vi "Purge uService from local lists.vi"(10 "Last Ack":refnum<class "Last Ack.lvclass">, 11 "Guardian in":refnum<class "Guardian.lvclass">) -> (0 "error out":errorcluster, 1 "uService ID":string, 2 "uService Properties":T1, 3 "Guardian out":refnum<class "Guardian.lvclass">)   [LabVIEW 2026, in "TALOS.lvlib" / "Guardian.lvlib" / "Guardian.lvclass"]
uses:
  Guardian.lvclass
  Classes/uService List/uService Properties.ctl
  builds/Actor Framework PPL/Actor Framework.lvlibp/1abvi3w/vi.lib/ActorFramework/Message Enqueuer/Message Enqueuer.lvclass
  C:/LabVIEW Code/TALOS/talos/Ancestor/Ancestor/Ancestor.lvclass
  builds/Actor Framework PPL/Actor Framework.lvlibp/1abvi3w/vi.lib/ActorFramework/LastAck/Last Ack.lvclass
  Classes/uService List/uService List.lvclass/uService List.ctl
  Ancestor/Ancestor/Ancestor.lvclass/Ancestor.ctl
  Classes/uService List/Get ID from Queue.vi
  Classes/uService List/Get Properties.vi
  Classes/uService List/Remove uService.vi
  Ancestor/Ancestor/Write uS List Ref.vi
  Ancestor/Ancestor/Read Distr uS Map ref.vi
  Ancestor/Ancestor/Read ID.vi
  Ancestor/Ancestor/Write Distr uS Map ref.vi
  Support VIs/Generate Error.vi
  FGV/Error Memory/Get Error Description.vi
  Support VIs/Get PC name.vi
  Support VIs/Get Class Name.vi
  <vilib>/Utility/error.llb/Clear Errors.vi
  FGV/Error Memory/Error Memory Core.vi
  <vilib>/AdvancedString/Delimited String to 1D String Array.vi
  <vilib>/AdvancedString/Delimited String to 1D String Array (string).vi
  Support VIs/Circus Root Path.vi
  FGV/Error Memory/Error Crt Lvl checker.vi
  FGV/Error Memory/Error Memory Core.vi/40c8088d-b597-4017-91af-faa98e00292e.vi
  FGV/Error Memory/Error Memory Core.vi/d4a3ab98-063c-4e44-b43d-fbdcfe6c2be2.vi
  Support VIs/Global Memory.vi
  <vilib>/Utility/LVClass/Get LV Class Name.vi
  Support VIs/Is in Packed Library.vi
  Support VIs/TALOS Root path.vi
  Support VIs/Read CSV worksheet.vi
  Support VIs/Global Constants.vi
  <vilib>/Utility/error.llb/General Error Handler.vi
  Support VIs/Error Log.vi
  Classes/uService List/uService List.lvclass
  Ancestor/Ancestor/Ancestor.lvclass
  <vilib>/Comparison/Equal/Equal Functor/Equal Functor.lvclass
  Classes/Distributed uService Map/Distributed uService Map.lvclass
  TALOS.lvlib
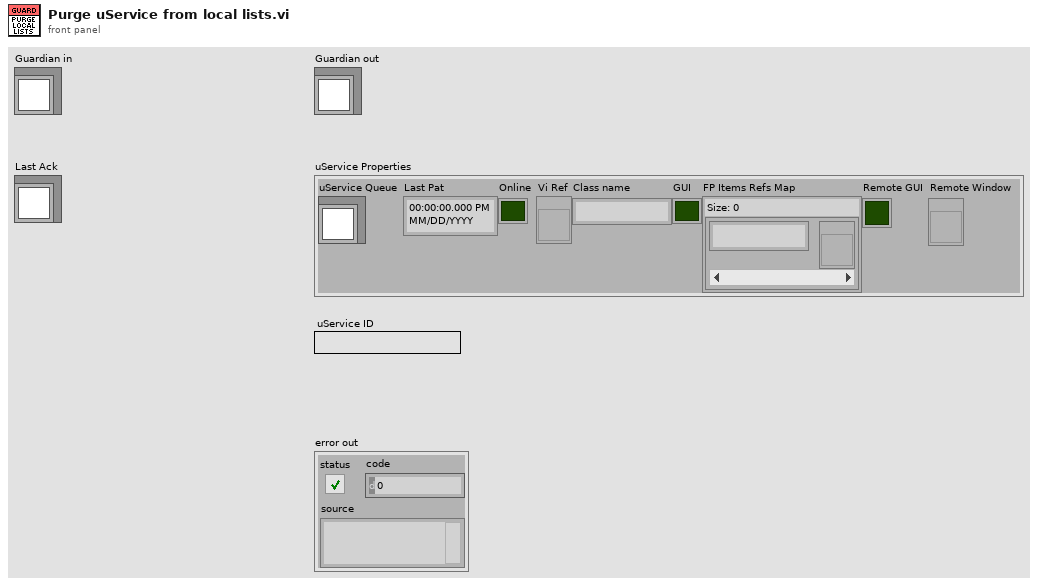
[diagram p1: front panel]
types:
  T1 = typedef "TALOS.lvlib/Classes.lvlib/uService List.lvclass/uService Properties.ctl" = cluster{"uService Queue":refnum<class "Message Enqueuer.lvclass">, "Last Pat":timestamp, "Online":bool, "Vi Ref":refnum<vi>, "Class name":string, "GUI":bool, "FP Items Refs Map":map{string, refnum<vi>}, "Remote GUI":bool, "Remote Window":refnum<vi>}
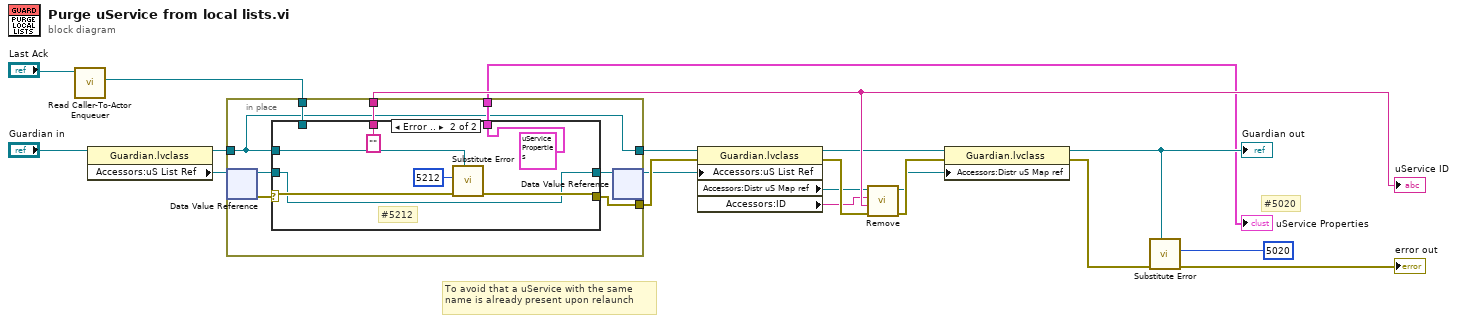
[diagram p0: block diagram]
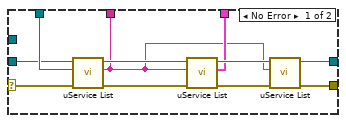
[diagram p2: hidden frame]
diagram:
  # "#5020"
  # "To avoid that a uService with the same name is already present upon relaunch"
  n1 = call "Read Caller-To-Actor Enqueuer.vi"("Last Ack"="Last Ack") -> ("Caller-to-Actor Enqueuer"=w17:refnum<class "Message Enqueuer.lvclass">)  [unwired: 10 in]
  n2 = property class="Guardian.lvclass"(reference="Guardian in") -> (reference out=w19:refnum<class "Guardian.lvclass">, "Accessors:uS List Ref"=w16:refnum<data-value>)  [unwired: 1 in, 1 out]
  n3 = in-place {
    in-place-border: w17 -> [w28]
    in-place-border: [w23] -> w20
    in-place-border: [w26] -> w8
    in-place-border: [w25] -> w1
    in-place-border: w19 -> [w21]
    in-place-border: [w21] -> w6
    n4 = in-place-dvr #1(w16) -> (w27:refnum<class "uService List.lvclass">, w22:errorcluster)
    n5 = case shown="Error .." w22 {
      selector: w22 -> [w29 w45]
      tunnel: w28 -> [w35 _]
      tunnel: w27 -> [w34 w41]
      tunnel: [w33 w43] -> w26
      tunnel: [w32 T1 {"uService Queue"=refnum, "Last Pat"=timestamp(0 s since 1904-01-01), "Online"=FALSE, "Vi Ref"=refnum, "Class name"="", "GUI"=FALSE, "FP Items Refs Map"={}, "Remote GUI"=FALSE, "Remote Window"=refnum} ("uService Properties")] -> w25
      tunnel: [w31 w41] -> w24
      tunnel: [w30 "" ("ID out")] -> w23
      tunnel: w21 -> [_ w44]
      frame No Error {
        n6 = call-poly "uService List.vi"("error in (no error)"=w29, "uService Queue"=w35, "uService List in"=w34) -> ("error out"=w36:errorcluster, "ID out"=w30:string, "uService List out"=w38:refnum<class "uService List.lvclass">)  [unwired: 6 in]
        n7 = call-poly "uService List.vi"("error in (no error)"=w36, "ID"=w30, "uService List in"=w38) -> ("error out"=w37:errorcluster, "uService Properties"=w32:T1, "uService List out"=w39:refnum<class "uService List.lvclass">)  [unwired: 6 in]
        n8 = call-poly "uService List.vi"("error in (no error)"=w37, "ID"=w30, "uService List in"=w39) -> ("error out"=w33:errorcluster, "uService List out"=w31:refnum<class "uService List.lvclass">)  [unwired: 7 in]
      }
      frame Error {
        # "#5212"
        n9 = call "Substitute Error.vi"("LabVIEW Object"=w44, "error in (no error)"=w45, "Error Code"=5212) -> ("error out"=w43:errorcluster)  [unwired: 8 in]
      }
    }
    n10 = in-place-dvr #1(w24) -> (w7:refnum<data-value>)  [unwired: 1 out]
  }
  "uService Properties" <- w1
  "uService ID" <- w20
  n11 = property class="Guardian.lvclass"(reference=w6, error in=w8, "Accessors:uS List Ref"=w7) -> (reference out=w12:refnum<class "Guardian.lvclass">, error out=w11:errorcluster, "Accessors:Distr uS Map ref"=w10:refnum<data-value>, "Accessors:ID"=w9:string)
  n12 = call "Remove.vi"("error in (no error)"=w11, "uService ID"=w20, "Guardian"=w9, "Distr uS Map ref in"=w10) -> ("error out"=w3:errorcluster, "Distr uS Map ref out"=w2:refnum<data-value>)  [unwired: 5 in, 1 out]
  n13 = property class="Guardian.lvclass"(reference=w12, error in=w3, "Accessors:Distr uS Map ref"=w2) -> (reference out=w5:refnum<class "Guardian.lvclass">, error out=w4:errorcluster)
  "Guardian out" <- w5
  n14 = call "Substitute Error.vi"("LabVIEW Object"=w5, "error in (no error)"=w4, "Error Code"=5020) -> ("error out"=→"error out":errorcluster)  [unwired: 8 in]
